vi "ttm_stop.vi"() -> (2 "creepRunningOut":bool)   [LabVIEW 2010]
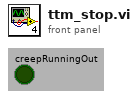
[diagram p1: front panel]
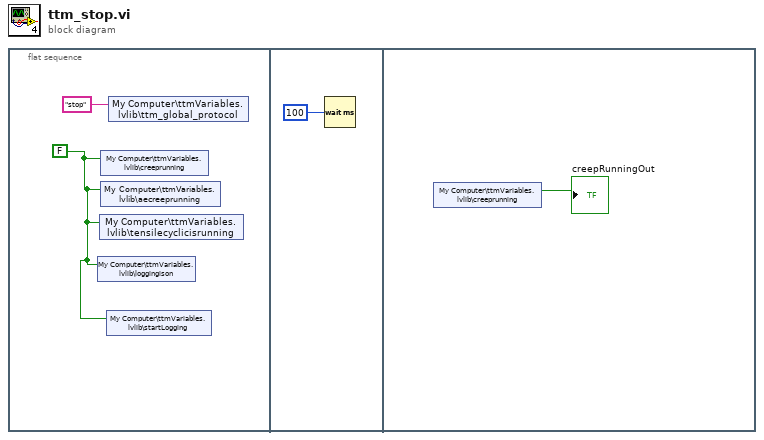
[diagram p0: block diagram]
diagram:
  n1 = flat-sequence {
    frame #0 {
      w1 = FALSE ("Busy")
      n2 = shared-variable "My Computer\\ttmVariables.lvlib\\loggingison"(w1) -> ()  [unwired: 1 in, 1 out]
      n3 = shared-variable "My Computer\\ttmVariables.lvlib\\tensilecyclicisrunning"(w1) -> ()  [unwired: 1 in, 1 out]
      n4 = shared-variable "My Computer\\ttmVariables.lvlib\\creeprunning"(w1) -> ()  [unwired: 1 in, 1 out]
      n5 = shared-variable "My Computer\\ttmVariables.lvlib\\aecreeprunning"(w1) -> ()  [unwired: 1 in, 1 out]
      n6 = shared-variable "My Computer\\ttmVariables.lvlib\\startLogging"(w1) -> ()  [unwired: 1 in, 1 out]
      n7 = shared-variable "My Computer\\ttmVariables.lvlib\\ttm_global_protocol"("stop" ("protocol")) -> ()  [unwired: 1 in, 1 out]
    }
    frame #1 {
      n8 = Wait (ms)(milliseconds to wait=u32 100) -> ()  [unwired: 1 out]
    }
    frame #2 {
      n9 = shared-variable "My Computer\\ttmVariables.lvlib\\creeprunning"() -> (→"creepRunningOut":bool)  [unwired: 1 in, 1 out]
    }
  }
